vi "test_Get Instrument Addon Name.vi"(8 "error in (no error)":errorcluster, 11 "TestCase in":refnum<class "Instrument Addon Scripting API Custom Device Unit Tests.lvclass">) -> (0 "error out":errorcluster, 3 "TestCase out":refnum<class "Instrument Addon Scripting API Custom Device Unit Tests.lvclass">)   [LabVIEW 2018, in "Instrument Addon Scripting API Custom Device Unit Tests.lvclass"]
uses:
  Instrument Addon Scripting API Custom Device Unit Tests.lvclass
  <vilib>/addons/_JKI Toolkits/VI Tester/TestCase.llb/TestCase.lvclass
  Instrument Addon Scripting API Test Assets/Instrument Addon Scripting API Test Assets.lvclass
  APIs/Scripting API/Instrument Addon Scripting API.lvlib
  C:/Program Files (x86)/National Instruments/LabVIEW 2018/vi.lib/addons/_JKI Toolkits/VI Tester/TestCase.llb/TestCase.lvclass
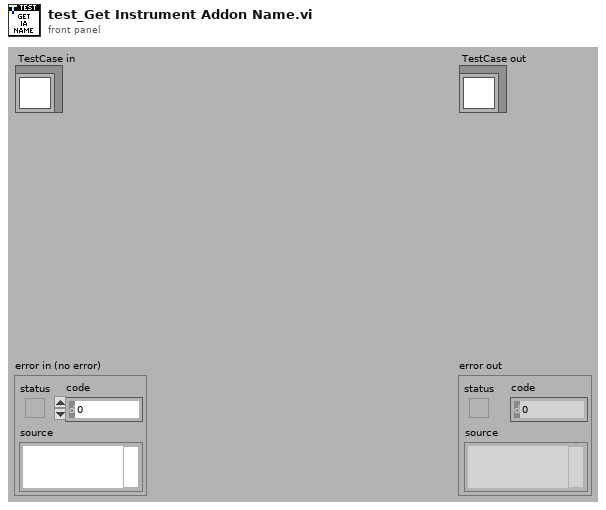
[diagram p1: front panel]
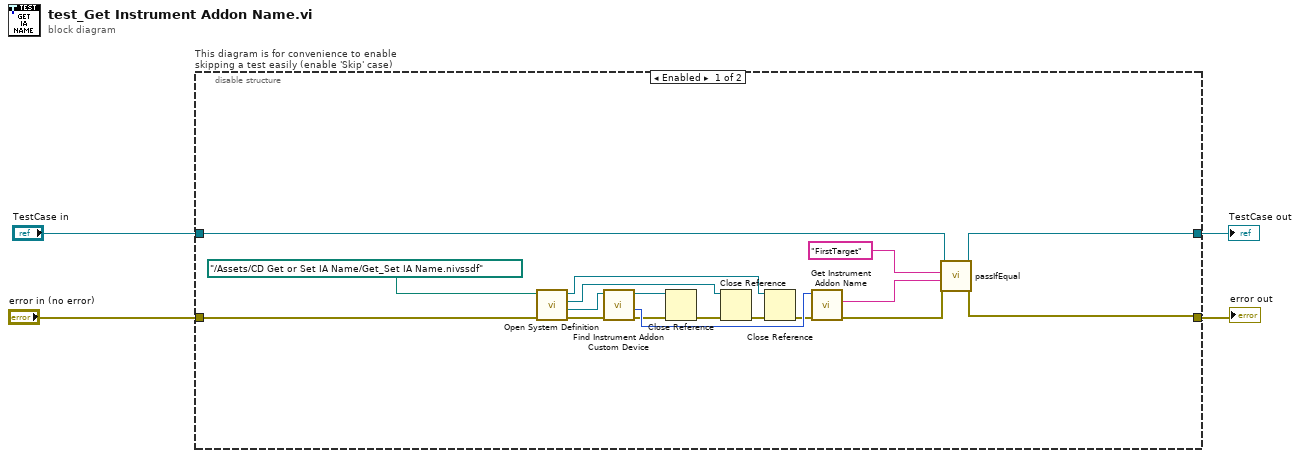
[diagram p0: block diagram]
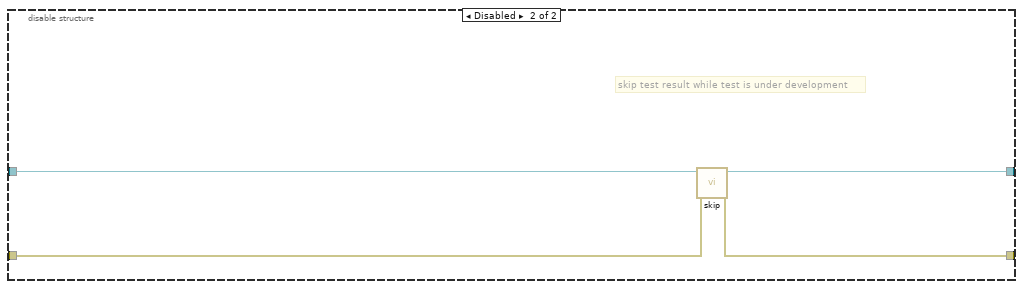
[diagram p2: hidden frame]
diagram:
  n1 = disable-structure "This diagram is for convenience to enable skipping a test easily (enable 'Skip' case)" shown="Enabled" {
    disable-tunnel: "TestCase in" -> [w22 w26]
    disable-tunnel: [w21 w24] -> w1
    disable-tunnel: [w20 w25] -> w3
    disable-tunnel: "error in (no error)" -> [w19 w23]
    frame Enabled {
      n2 = call "Open System Definition.vi"("error in (no error)"=w19, "System Definition File"=path "../Assets/CD Get or Set IA Name/Get_Set IA Name.nivssdf") -> ("error out"=w18:errorcluster, "Target Refnum"=w17:refnum<k24>, "Root Refnum"=w9:refnum<k24>, "System Definition Refnum"=w10:refnum<k24>)  [unwired: 6 in]
      n3 = call "Find Instrument Addon Custom Device.vi"("error in"=w18, "target in"=w17) -> ("error out"=w6:errorcluster, "NodeID"=w16:u64, "target out"=w7:refnum<k24>)  [unwired: 7 in]
      n4 = Close Reference(reference=w7, error in (no error)=w6) -> (error out=w8:errorcluster)
      n5 = Close Reference(reference=w9, error in (no error)=w8) -> (error out=w11:errorcluster)
      n6 = Close Reference(reference=w10, error in (no error)=w11) -> (error out=w5:errorcluster)
      n7 = call "Get Instrument Addon Name.vi"("Error In"=w5, "Instrument Addon Refnum In"=w16) -> ("Error Out"=w13:errorcluster, "Name"=w14:string)  [unwired: 7 in, 1 out]
      n8 = call-dynamic "passIfEqual.vi"("error in (no error)"=w13, "y"=w14, "x"="FirstTarget", "TestCase in"=w22) -> ("error out"=w20:errorcluster, "TestCase out"=w21:refnum<class "Instrument Addon Scripting API Custom Device Unit Tests.lvclass">)  [unwired: 6 in]
    }
    frame Disabled {
      # "skip test result while test is under development"
      n9 = call <vilib>:"skip.vi"("error in (no error)"=w23, "TestCase in"=w26) -> ("error out"=w25:errorcluster, "TestCase out"=w24:refnum<class "Instrument Addon Scripting API Custom Device Unit Tests.lvclass">)  [unwired: 8 in]
    }
  }
  "error out" <- w3
  "TestCase out" <- w1
